vi "NameToTag.vi"(11 "String":string) -> (3 "tag":T1)   [LabVIEW 2018, in "MasterProgramSupportFunctions.lvlib"]
uses:
  MasterProgramSupportFunctions.lvlib
  VI_tags.ctl
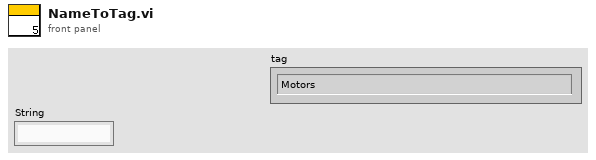
[diagram p1: front panel]
types:
  T1 = typedef "MasterProgramSupportFunctions.lvlib/VI_tags.ctl" = enum16{"Motors", "Gage", "Tektro3107", "XimeaMainCamera", "ContinuousMainScan"}
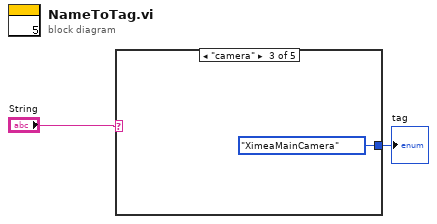
[diagram p0: block diagram]
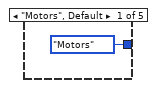
[diagram p2: hidden frame]
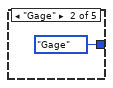
[diagram p3: hidden frame]
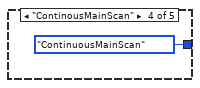
[diagram p4: hidden frame]
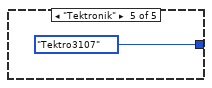
[diagram p5: hidden frame]
diagram:
  n1 = case shown="\"camera\"" "String" {
    tunnel: [VI_tags."Motors" ("Enum") VI_tags."Gage" ("Enum") VI_tags."XimeaMainCamera" ("Enum") VI_tags."ContinuousMainScan" ("Enum") VI_tags."Tektro3107" ("Enum")] -> w1
    frame "Motors", Default {
    }
    frame "Gage" {
    }
    frame "camera" {
    }
    frame "ContinousMainScan" {
    }
    frame "Tektronik" {
    }
  }
  "tag" <- w1
